vi "Remove_FF_lone_spikes.vi"(3 "ADC Frequency Hz":dbl=1000.0 format="%.2f", 4 "Bkgnd variance":dbl format="%.6f", 5 "AIC index":i32, 6 "Time Trace":dbl[](array[numeric])) -> (0 "No Removed":i32, 2 "Filtered Time Trace":dbl[](array[numeric]))   [LabVIEW 2012]
uses:
  Globals/Meas_global.vi
  <vilib>/Analysis/NI_AALBase.lvlib
panel:
  out "Spike must be greater than":dbl
  out "Waveform Graph":dbl[][](graph)
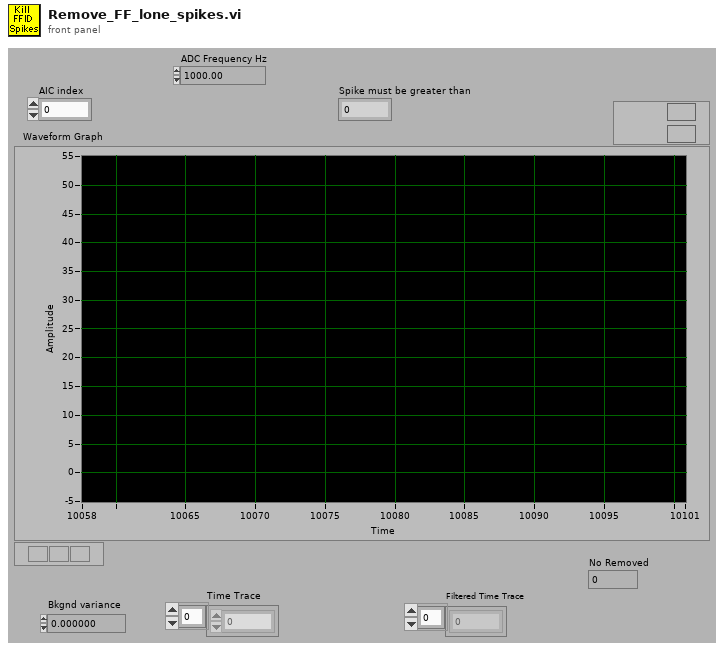
[diagram p1: front panel]
types:
  T1 = typedef "Analysis_info_cluster.ctl" = cluster{"Colour":u32, "Inst type":T2, "Inst name":string, "Symbol":string, "Code name":string, "Extra Info":string, "Inst Array":T3, "Extra Titles":string[], "Extra Values":string[], "U":dbl, "u^2":dbl, "u^3":dbl, "u^4":dbl, "Skew_u":dbl, "Kurt_u":dbl, "Sd Error in Mean":dbl, "% u'/U":dbl, "X":dbl, "Y":dbl, "Z":dbl, "Timescale integral to 25%":dbl, "Sd Error in Variance":dbl, "Calib File":path, "Calib Constants":dbl[], "Output Position":bool, "Full Stats":bool, "Av Sampling Rate":dbl, "Av No of Samples":dbl, "Total Meas Time (s)":dbl, "ADAM Ch Name":string}
  T2 = typedef "Inst_type.ctl" = enum16{"Propeller anemometer", "Raw voltage", "Pressure Transducer", "Pitot-static tube", "Preston tube", "Hot wire", "Cross wire 1", "Cross wire 2", "Generic Linear", "Generic Polynomial", "Generic BackPoly", "Fast FID", "Thermocouple", "Cold wire", "Pulsed Wire", "LDA Vel", "LDA Tran time", "LDA Arr time"}
  T3 = typedef "Instrument_Array.ctl" = enum16{"PWA", "LDA", "Analogue"}
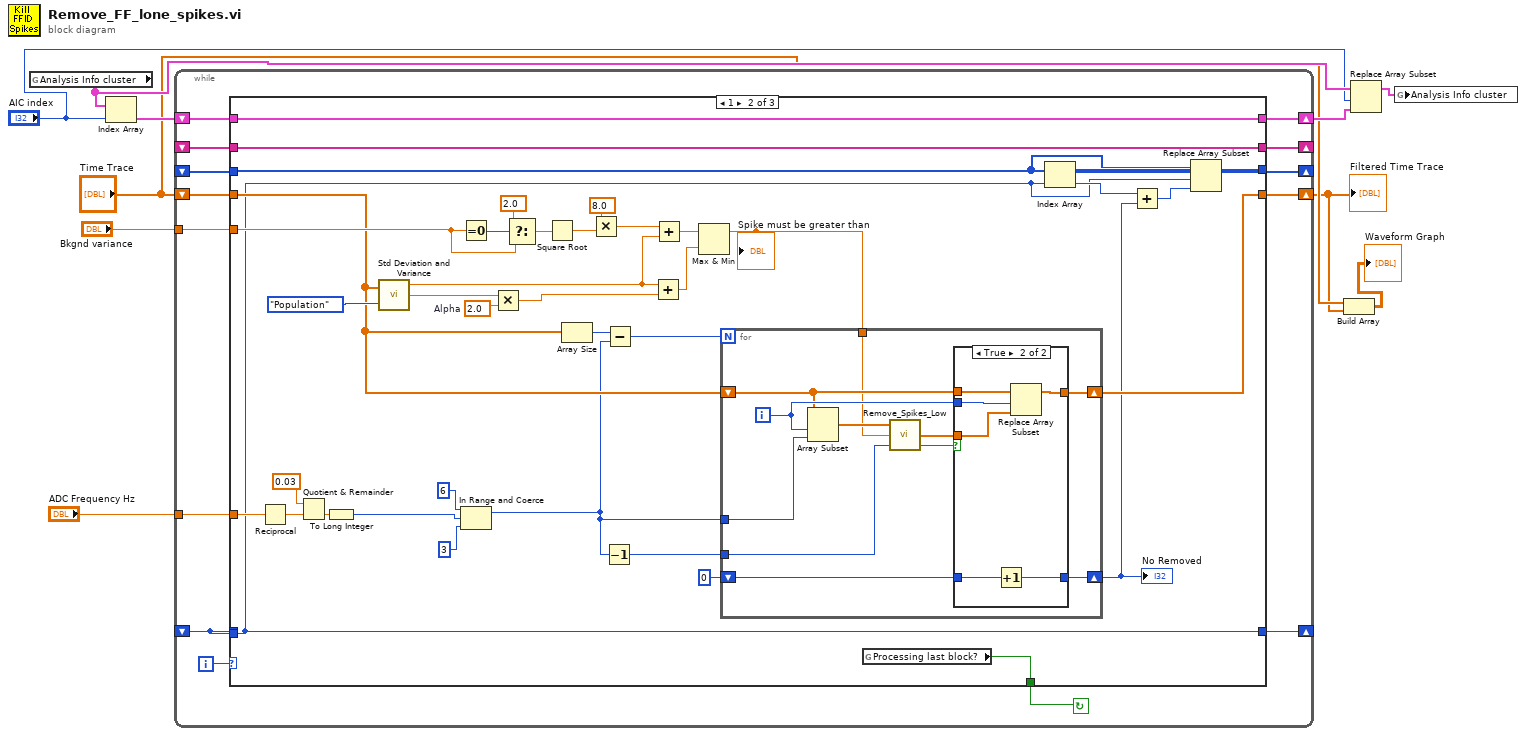
[diagram p0: block diagram]
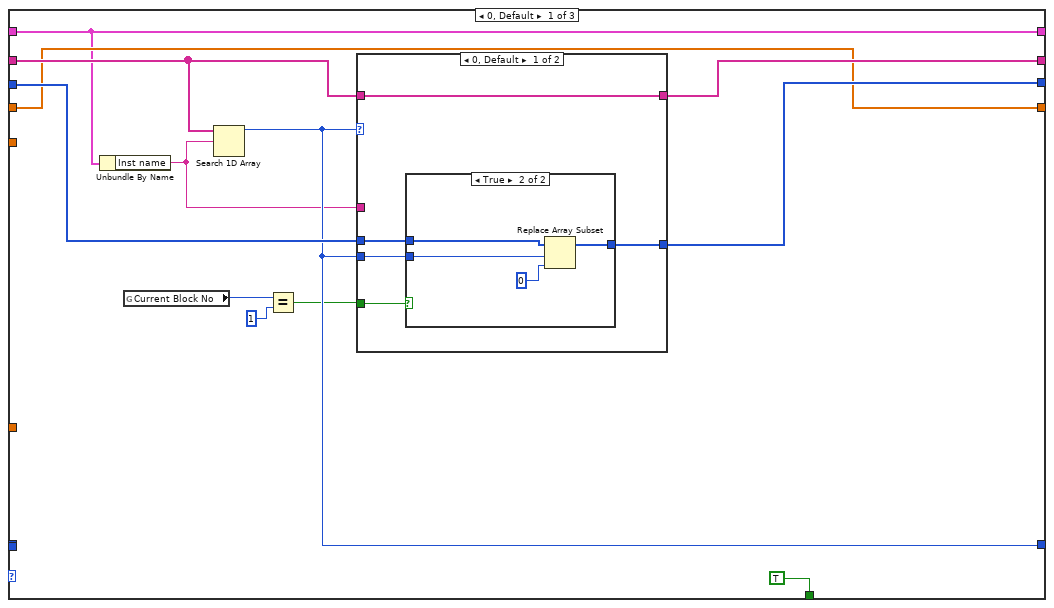
[diagram p2: hidden frame]
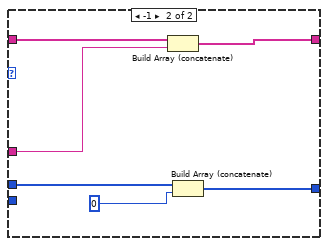
[diagram p4: hidden frame]
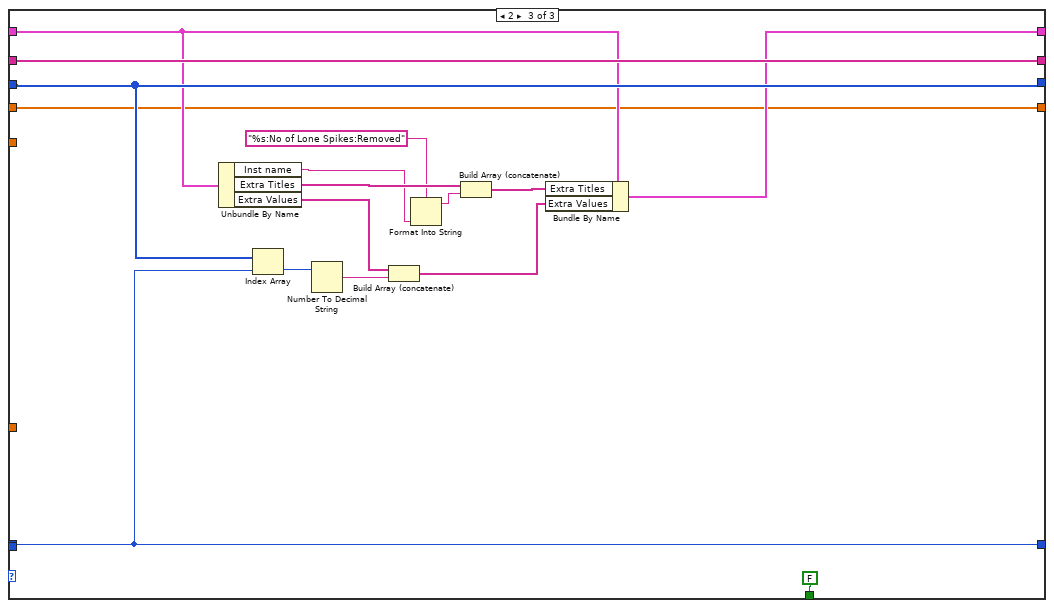
[diagram p6: hidden frame]
diagram:
  n1 = global read "Meas_global.vi" "Analysis Info cluster"() -> (w7:T1[])
  n2 = Index Array(array=w7, index="AIC index") -> (element=w8:T1)
  n3 = while {
    shift-left: _ -> [w21]
    shift-right: [w23] -> _
    shift-right: [w19] -> _
    shift-left: _ -> [w20]
    shift-right: [w17] -> _
    shift-left: _ -> [w18]
    shift-right: [w15] -> w6
    shift-left: w8 -> [w16]
    tunnel: "Bkgnd variance" -> [w14]
    shift-right: [w12] -> w2
    shift-left: "Time Trace" -> [w13]
    tunnel: "ADC Frequency Hz" -> [w11]
    i -> [w24]
    stop <- w22 continue-if-true
    n4 = case shown="1" w24 {
      tunnel: [w29 w67 w123] -> w23
      tunnel: [TRUE w65 FALSE ("Processing last block?")] -> w22
      tunnel: w21 -> [_ _ w123]
      tunnel: w21 -> [_ w67 _]
      tunnel: w20 -> [w33 w83 w121]
      tunnel: [w32 w83 w121] -> w19
      tunnel: w18 -> [w31 w82 w120]
      tunnel: [w30 w80 w120] -> w17
      tunnel: w16 -> [w26 w79 w117]
      tunnel: [w26 w79 w119] -> w15
      tunnel: w14 -> [_ w78 _]
      tunnel: w13 -> [w27 w71 w113]
      tunnel: [w27 w66 w113] -> w12
      tunnel: w11 -> [_ w76 _]
      frame 0, Default {
        n5 = Unbundle By Name(w26) -> ("Inst name"=w25:string)
        n6 = global read "Meas_global.vi" "Current Block No"() -> (w35:i32)
        n7 = Search 1D Array(1D array=w33, element=w25) -> (index of element=w29:i32)  [unwired: 1 out]
        n8 = Equal?(x=w35, y=1) -> (x = y?=w28:bool)
        n9 = case shown="0, Default" w29 {
          tunnel: w33 -> [w41 w52]
          tunnel: w25 -> [_ w51]
          tunnel: [w41 w50] -> w32
          tunnel: w31 -> [w40 w49]
          tunnel: [w39 w48] -> w30
          tunnel: w29 -> [w38 _]
          tunnel: w28 -> [w37 _]
          frame 0, Default {
            n10 = case shown="True" w37 {
              tunnel: w40 -> [w42 w46]
              tunnel: [w42 w45] -> w39
              tunnel: w38 -> [_ w44]
              frame False {
              }
              frame True {
                n11 = Replace Array Subset(array=w46, new element=0, index=w44) -> (w45:i32[])
              }
            }
          }
          frame -1 {
            n12 = Build Array (concatenate)(w52, w51) -> (w50:string[])
            n13 = Build Array (concatenate)(w49, 0) -> (w48:i32[])
          }
        }
      }
      frame 1 {
        w59 = 2.0  # Alpha
        n14 = Reciprocal(x=w76) -> (1/x=w74:dbl)
        n15 = Quotient & Remainder(x=0.03, y=w74) -> (floor(x/y)=w73:dbl)  [unwired: 1 out]
        n16 = To Long Integer(number=w73) -> (32bit integer=w53:i32)
        n17 = call <vilib>:"Std Deviation and Variance.vi"("X"=w71, "Weighting (Sample)"=enum16{"Sample", "Population"}."Population") -> ("mean"=w61:dbl, "standard deviation"=w60:dbl)  [unwired: 1 out]
        n18 = Equal To 0?(x=w78) -> (x = 0?=w89:bool)
        n19 = In Range and Coerce(upper limit=6, x=w53, lower limit=3) -> (coerced(x)=w54:i32)  [unwired: 1 out]
        n20 = Multiply(x=w60, y=w59) -> (x*y=w62:dbl)
        n21 = Select(t=2.0, s=w89, f=w78) -> (s? t:f=w87:dbl)
        n22 = Square Root(x=w87) -> (sqrt(x)=w58:dbl)
        n23 = Array Size(array=w71) -> (size(s)=w70:i32)
        n24 = Multiply(x=8.0 ("y"), y=w58) -> (x*y=w90:dbl)
        n25 = Decrement(x=w54) -> (x-1=w72:i32)
        n26 = Subtract(x=w70, y=w54) -> (x-y=w69:i32)
        n27 = Add(x=w61, y=w62) -> (x+y=w84:dbl)
        n28 = Add(x=w90, y=w61) -> (x+y=w85:dbl)
        n29 = Max & Min(x=w85, y=w84) -> (max(x,y)=w68:dbl)  [unwired: 1 out]
        "Spike must be greater than" <- w68
        n30 = for {
          N: w69 -> [_]
          shift-right: [w94] -> w66
          shift-left: w71 -> [w95]
          tunnel: w54 -> [w101]
          tunnel: w72 -> [w100]
          tunnel: w68 -> [w93]
          shift-right: [w92] -> w64
          shift-left: 0 -> [w91]
          i -> [w97]
          n31 = Array Subset(array=w95, index=w97, length=w101) -> (w99:dbl[])
          n32 = call "Remove_Spikes_Low.vi"("index"=w100, "Background noise"=w93, "Time Trace"=w99) -> ("Spike"=w98:bool, "Filtered Time Trace"=w96:dbl[])  [unwired: 1 out]
          n33 = case shown="True" w98 {
            tunnel: w97 -> [_ w109]
            tunnel: w96 -> [_ w108]
            tunnel: w95 -> [w103 w107]
            tunnel: [w103 w106] -> w94
            tunnel: [w102 w104] -> w92
            tunnel: w91 -> [w102 w105]
            frame False {
            }
            frame True {
              n34 = Increment(x=w105) -> (x+1=w104:i32)
              n35 = Replace Array Subset(array=w107, new element=w108, index=w109) -> (w106:dbl[])
            }
          }
        }
        "No Removed" <- w64
        n36 = global read "Meas_global.vi" "Processing last block?"() -> (w65:bool)
        n37 = Index Array(array=w82, index=w67) -> (element=w81:i32)
        n38 = Add(x=w81, y=w64) -> (x+y=w77:i32)
        n39 = Replace Array Subset(array=w82, new element=w77, index=w67) -> (w80:i32[])
      }
      frame 2 {
        n40 = Unbundle By Name(w117) -> ("Inst name"=w111:string, "Extra Titles"=w116:string[], "Extra Values"=w115:string[])
        n41 = Index Array(array=w120, index=w123) -> (element=w122:i32)
        n42 = Number To Decimal String(number=w122) -> (decimal integer string=w124:string)  [unwired: 1 out]
        n43 = Build Array (concatenate)(w115, w124) -> (w114:string[])
        n44 = Format Into String(format string="%s:No of Lone Spikes:Removed", w111) -> (resulting string=w112:string)  [unwired: 2 in, 1 out]
        n45 = Build Array (concatenate)(w116, w112) -> (w118:string[])
        n46 = Bundle By Name(cluster=w117, "Extra Titles"=w118, "Extra Values"=w114) -> (w119:T1)
      }
    }
  }
  "Filtered Time Trace" <- w2
  n47 = Build Array("Time Trace", w2) -> (→"Waveform Graph":dbl[][])
  n48 = Replace Array Subset(array=w7, new element=w6, index="AIC index") -> (w4:T1[])
  n49 = global write "Meas_global.vi" "Analysis Info cluster"(w4) -> ()
